vi "Insertar SubPanel-Modificado.vi"(8 "error in (no error)":errorcluster, 10 "VI Ref":refnum<vi>, 11 "Subpanel Ref":refnum<vi>) -> (0 "error out":errorcluster)   [LabVIEW 2020]
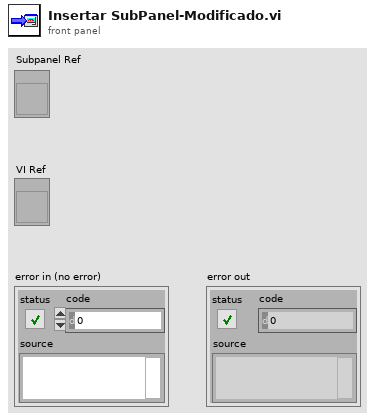
[diagram p1: front panel]
types:
  T1 = enum32{"Invalid", "Standard", "Closed", "Hidden", "Minimized", "Maximized"}
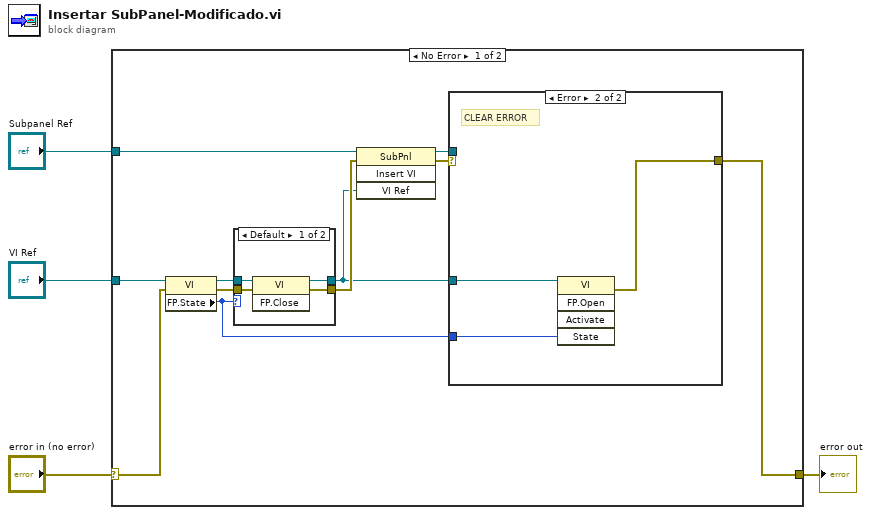
[diagram p0: block diagram]
diagram:
  n1 = case shown="No Error" "error in (no error)" {
    selector: "error in (no error)" -> [w8 w26]
    tunnel: "VI Ref" -> [w15 _]
    tunnel: "Subpanel Ref" -> [w6 _]
    tunnel: [w7 w26] -> w1
    frame No Error {
      n2 = property class="VI"(reference=w15, error in=w8) -> (reference out=w14:refnum<vi>, error out=w13:errorcluster, "FP.State"=w5:T1)
      n3 = case shown="Default" w5 {
        tunnel: w14 -> [w19 w21]
        tunnel: w13 -> [w18 w20]
        tunnel: [w17 w21] -> w9
        tunnel: [w16 w20] -> w12
        frame Default {
          n4 = invoke class="VI" method="FP.Close"(reference=w19, error in=w18) -> (reference out=w17:refnum<vi>, error out=w16:errorcluster)  [unwired: 1 in, 1 out]
        }
        frame "Closed" {
        }
      }
      n5 = invoke class="SubPnl" method="Insert VI"(reference=w6, error in=w12, "VI Ref"=w9) -> (reference out=w10:refnum<vi>, error out=w11:errorcluster)  [unwired: 1 in, 2 out]
      n6 = case shown="Error" w11 {
        selector: w11 -> [w22 _]
        tunnel: w10 -> [_ _]
        tunnel: w9 -> [_ w25]
        tunnel: w5 -> [_ w23]
        tunnel: [w22 w24] -> w7
        frame No Error {
        }
        frame Error {
          # "CLEAR ERROR"
          n7 = invoke class="VI" method="FP.Open"(reference=w25, "State"=w23) -> (error out=w24:errorcluster)  [unwired: 3 in, 4 out]
        }
      }
    }
    frame Error {
    }
  }
  "error out" <- w1
